vi "Log.vi"(7 "Local Variables":T2={"Core"={"Current VI"=refnum, "Close Panel on Exit?"=FALSE, "VI Name"="", "VI Path"=path ""}, "Lof File Ref"=refnum, "Log?"=FALSE, "Logging Level"=enum."Debug", "Current Case"="", "Shared Variable Address"="", "reader endpoint"="", "writer endpoint"="", "Detected Systems"=[], "Dataset"={"System Status"={"Power On Off"=FALSE, "Discharge Temp"=0.0, "Liquid Temp"=0.0, "Suction Temp"=0.0, "Ambient Temp"=0.0, "Sleep"=FALSE, "System Status"=enum."Sleep", "M1 Actuated"=FALSE, "M2 Actuated"=FALSE, "Sleep Timer"=0.0, "M1 Bin"={"Bin String"="", "Bin Color"=enum."White"}, "M2 Bin"={"Bin String"="", "Bin Color"=enum."White"}, "Discharge Pressure"=0.0, "Suction Pressure"=0.0, "Compression Ratio"=0.0, "Compressor Amps"=0.0, "Compressor Hours"=0.0, "Bypass Steps"=0, "SubCooling"=0.0, "SuperHeat"=0.0, "Serial Number"="", "EMO detected"=FALSE, "EMO Tripped"=FALSE, "Thermal cutoff"=FALSE, "Thermal cutoff 2"=FALSE, "High Pressure switch"=FALSE, "Running Time"=timestamp(0 s since 1904-01-01), "SOM Status"={"Boot Up Time"=timestamp(0 s since 1904-01-01), "Software Version"="", "CPU Usage"=0.0, "Memory Available"=0.0, "SD card free space"=0.0, "SOM Storage"=0.0}, "Cascade Extra"={"Discharge Temp High Side"=0.0, "Suction Temp High Side"=0.0, "Liquid Temp High side"=0.0, "Discharge Pressure 2"=0.0, "Suction Pressure 2"=0.0, "Low Side RPM"=0.0, "High Side RPM"=0.0}}, "M1 Status"={"Case Temp"=0.0, "Evap Temp"=0.0, "Heater %"=0.0, "EEV Steps"=0, "Set Temp"=0.0, "Feedback"=0, "Power Drive"=FALSE, "Piston Volts"=0.0, "Safe Temp"=FALSE, "Power"=FALSE, "Thermal State"=enum."Ramp Up", "Error"=FALSE, "In tollerance"=FALSE, "Head State"=enum."Disabled", "Piston Force"=0.0, "Package"="", "Dynamic SV"=0.0, "PV"=0.0, "TSD Temp"=0.0, "DC Load Watts"=0.0, "AC Load Watts"=0.0, "Intec Feedback"=0.0}, "M2 Status"={"Case Temp"=0.0, "Evap Temp"=0.0, "Heater %"=0.0, "EEV Steps"=0, "Set Temp"=0.0, "Feedback"=0, "Power Drive"=FALSE, "Piston Volts"=0.0, "Safe Temp"=FALSE, "Power"=FALSE, "Thermal State"=enum."Ramp Up", "Error"=FALSE, "In tollerance"=FALSE, "Head State"=enum."Disabled", "Piston Force"=0.0, "Package"="", "PV"=0.0, "Dynamic SV"=0.0, "TSD"=0.0, "AC Load Watts"=0.0}, "Config Data"={"Packages"={"DUT Force lbf"={" 0"=0, " 1"=0, " 2"=0, "3"=0, "4"=0, "5"=0, " 6"=0, "7"=0, "8"=0, "9"=0}, "DUT Names"={"0"="", "1"="", "2"="", "3"="", "4"="", "5"="", "6"="", "7"="", "8"="", "9"=""}}, "Heater PID"={"P"=0.0, "I"=0.0, "D"=0.0}, "Piston Settings"={"Forces Slope"=0.0, "Forces Intercept"=0.0, "Transition Force"=0.0, "Up Force"=0.0, "Diameter (mm)"=0.0, "Delay (ms)"=0.0, "Pressure Ramp Delay (ms)"=0.0}, "Safe Temps"={"Minimum"=17, "Enabled"=TRUE, "Maximum"=95}, "System Settings"={"Number of Heads"=0, "60Hz Power"=TRUE, "FTC200"=TRUE, "AutoStartup"=FALSE, "Purge"=TRUE, "Sensors"=TRUE, "HandClamp"=TRUE, "ATE"=TRUE, "Benchtop"=TRUE, "Production"=TRUE, "Refrigerant"=enum."r404a", "Handler"=TRUE, "Shuttle"=TRUE, "220V"=FALSE, "Cascade"=FALSE, "Suction Sensor"=enum."YCQB02H01", "Discharge Sensor"=enum."YCQB05H01"}, "Stepper Settings "={"Microstepping"=enum."Full", "Velocity"=8}, "Set Point Range"={"Max"=0.0, "Min"=0.0}, "Pedestal Check DeltaT"=0.0, "Ramp Delta T"=0.0, "Ramp-SS Threshold"=0.0, "SS Tolerance"=0.0, "EEV PID"={"Ramp Up Target"=0.0, "Ramp Down Target"=0.0, "Steady State Target"=0.0, "Output"={"Max"=0.0, "Min"=0.0}, "EBB and Flow Temp TH"=0.0, "Cryomode EEV Max"=0.0, "Valve minimum opening "=0.0, "Ramp Up EEV Steps"=0.0, "Ramp Down EEV Steps"=0.0, "SS EEV Steps Reset"=0.0, "EBB and Flow Tol"=0.0, "Gains"={"P"=0.0, "I"=0.0, "D"=0.0}, "Dissabled Target"=0.0, "CryoMode Gains"={"P"=0.0, "I"=0.0, "D"=0.0}, "M1 SuperHeat Setpoint"=0.0, "M2 Gains"={"P"=0.0, "I"=0.0, "D"=0.0}, "Flow Curve"=enum.""}, "Sleep Timeout"=0.0, "Bypass Values"={"Bypass Valve"=TRUE, "Flow Curve"=enum."0", "Output"={"Max"=0, "Min"=0}, "Feedback"=enum."Temperature", "Cyth Bypass"=TRUE, "PID"={"P"=0.0, "I"=0.0, "D"=0.0}, "Pressure setpoint"=0, "Cryo Temp"=0, "Superheat Setpoint"=0, "Cryo Setpoint"=0}, "Default Temp"=0.0, "InTEC"={"Enabled"=FALSE, "IP"="192.168.1.100", "Port"=5000}, "M1 TSD"={"Gain"=0.0, "Offset"=0.0, "V Offset "=0.0}, "M2 TSD"={"Gain"=0.0, "Offset"=0.0, "V Offset "=0.0}, "M1 T-Case Calibration"={"Gain"=0.0, "Offset"=0.0}, "M2 T-Case Calibration"={"Gain"=0.0, "Offset"=0.0}, "Heater PID TSD"={"P"=0.0, "I"=0.0, "D"=0.0}, "M2 Heater PID"={"P"=0.0, "I"=0.0, "D"=0.0}}}, "Network Data Down"={"M1 Commands"={"Set Temp"=20.0, "Power Drive"=FALSE, "Feedback"=1, "Package"=0, "Enable"=FALSE}, "M2 Commands"={"Set Temp"=20.0, "Power Drive"=FALSE, "Feedback"=1, "Package"=0, "Enable"=FALSE}, "System Power On Off"=FALSE, "New Data"=enum."M1 Set Point", "Stop RT"=FALSE, "Config Data"={"Packages"={"DUT Force lbf"={" 0"=0, " 1"=0, " 2"=0, "3"=0, "4"=0, "5"=0, " 6"=0, "7"=0, "8"=0, "9"=0}, "DUT Names"={"0"="", "1"="", "2"="", "3"="", "4"="", "5"="", "6"="", "7"="", "8"="", "9"=""}}, "Heater PID"={"P"=0.0, "I"=0.0, "D"=0.0}, "Piston Settings"={"Forces Slope"=0.0, "Forces Intercept"=0.0, "Transition Force"=0.0, "Up Force"=0.0, "Diameter (mm)"=0.0, "Delay (ms)"=0.0, "Pressure Ramp Delay (ms)"=0.0}, "Safe Temps"={"Minimum"=17, "Enabled"=TRUE, "Maximum"=95}, "System Settings"={"Number of Heads"=0, "60Hz Power"=TRUE, "FTC200"=TRUE, "AutoStartup"=FALSE, "Purge"=TRUE, "Sensors"=TRUE, "HandClamp"=TRUE, "ATE"=TRUE, "Benchtop"=TRUE, "Production"=TRUE, "Refrigerant"=enum."r404a", "Handler"=TRUE, "Shuttle"=TRUE, "220V"=FALSE, "Cascade"=FALSE, "Suction Sensor"=enum."YCQB02H01", "Discharge Sensor"=enum."YCQB05H01"}, "Stepper Settings "={"Microstepping"=enum."Full", "Velocity"=8}, "Set Point Range"={"Max"=0.0, "Min"=0.0}, "Pedestal Check DeltaT"=0.0, "Ramp Delta T"=0.0, "Ramp-SS Threshold"=0.0, "SS Tolerance"=0.0, "EEV PID"={"Ramp Up Target"=0.0, "Ramp Down Target"=0.0, "Steady State Target"=0.0, "Output"={"Max"=0.0, "Min"=0.0}, "EBB and Flow Temp TH"=0.0, "Cryomode EEV Max"=0.0, "Valve minimum opening "=0.0, "Ramp Up EEV Steps"=0.0, "Ramp Down EEV Steps"=0.0, "SS EEV Steps Reset"=0.0, "EBB and Flow Tol"=0.0, "Gains"={"P"=0.0, "I"=0.0, "D"=0.0}, "Dissabled Target"=0.0, "CryoMode Gains"={"P"=0.0, "I"=0.0, "D"=0.0}, "M1 SuperHeat Setpoint"=0.0, "M2 Gains"={"P"=0.0, "I"=0.0, "D"=0.0}, "Flow Curve"=enum.""}, "Sleep Timeout"=0.0, "Bypass Values"={"Bypass Valve"=TRUE, "Flow Curve"=enum."0", "Output"={"Max"=0, "Min"=0}, "Feedback"=enum."Temperature", "Cyth Bypass"=TRUE, "PID"={"P"=0.0, "I"=0.0, "D"=0.0}, "Pressure setpoint"=0, "Cryo Temp"=0, "Superheat Setpoint"=0, "Cryo Setpoint"=0}, "Default Temp"=0.0, "InTEC"={"Enabled"=FALSE, "IP"="192.168.1.100", "Port"=5000}, "M1 TSD"={"Gain"=0.0, "Offset"=0.0, "V Offset "=0.0}, "M2 TSD"={"Gain"=0.0, "Offset"=0.0, "V Offset "=0.0}, "M1 T-Case Calibration"={"Gain"=0.0, "Offset"=0.0}, "M2 T-Case Calibration"={"Gain"=0.0, "Offset"=0.0}, "Heater PID TSD"={"P"=0.0, "I"=0.0, "D"=0.0}, "M2 Heater PID"={"P"=0.0, "I"=0.0, "D"=0.0}}, "TTV Test"=FALSE, "Profile Test"=FALSE}, "IP Address"="", "Network Connection"=FALSE, "URI Directory"="", "File list in SoM"=[], "System State"=enum."Idle", "TTV Test"={"Power Seq"=[], "PS Connection"=FALSE, "OutputState"=FALSE, "Step"=0, "Current Cycle"=0}, "Profile"={"Profile Temp"=FALSE, "Profile Info"={"Start Temp"=0.0, "End Temp"=0.0, "Duration"=0.0, "dt"=0.0, "Iteration"=0}, "Current Cycle"=0}, "M1 Original Temps"=[], "M1 Mean Temps"=[], "M2 Original Temps"=[], "M2 Mean Temps"=[]} {"M2 Mean Temps" format="%#_13g"; "M2 Original Temps" format="%#_13g"; "M1 Mean Temps" format="%#_13g"; "M1 Original Temps" format="%#_13g"; "Profile"."Profile Info"."dt" format="%<%H:%M:%S>t"; "Profile"."Profile Info"."Duration" format="%<%H:%M:%S>t"; "Network Data Down"."M1 Commands"."Package" items=["CNF75XX", "CN73XX", "CN78XX", "CN88XX"]; "Network Data Down"."M1 Commands"."Feedback" items=["Evap Temp", "Case Temp"]; "Network Data Down"."M2 Commands"."Package" items=["CNF75XX", "CN73XX", "CN78XX", "CN88XX"]; "Network Data Down"."M2 Commands"."Feedback" items=["Evap Temp", "Case Temp"]; "Dataset"."System Status"."SOM Status"."Boot Up Time" format="%<%x %.3X>T"; "Dataset"."System Status"."Running Time" format="%<%x %.3X>T"; "Dataset"."M1 Status"."Feedback" items=["Evap Temp", "Case Temp", "Intec Temp", "TSD  Temp", "Autotune", "Extra"]; "Dataset"."M2 Status"."Feedback" items=["Evap Temp", "Case Temp"]}, 8 "error in (no error)":errorcluster, 11 "Log Level":T1) -> (0 "error out":errorcluster)   [LabVIEW 2019, in "GUI.lvlib"]
uses:
  GUI.lvlib
  Public Controls/GUI Variables.ctl
  Public Controls/Full Dataset.ctl
  Public Controls/Network Data Down.ctl
  Public Controls/Power Sequence.ctl
  Private Controls/Log Level.ctl
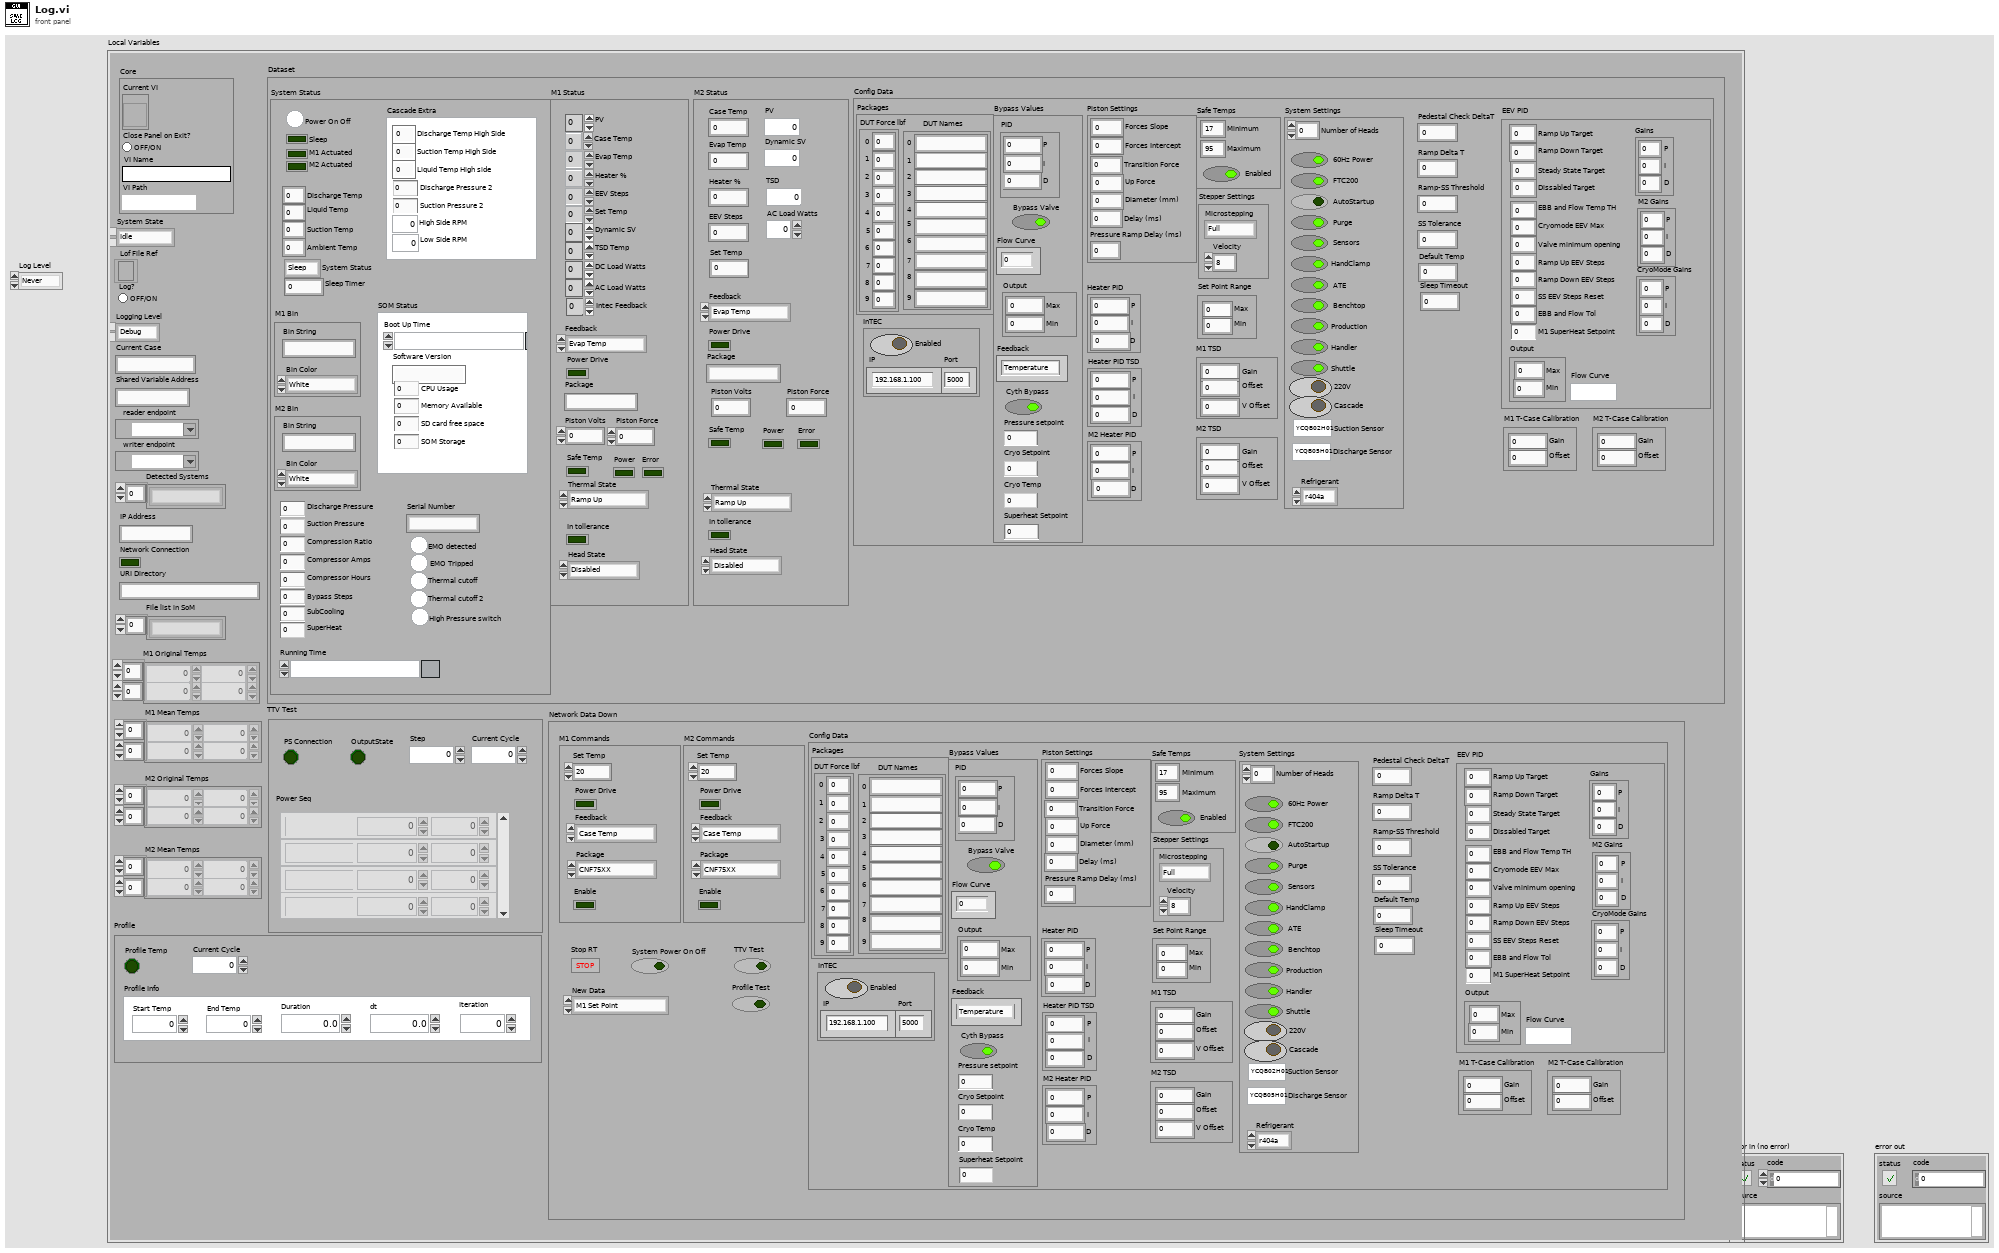
[diagram p1: front panel]
types:
  T1 = typedef "GUI.lvlib/Log Level.ctl" = enum16{"Never", "Debug", "Info", "Critical"}
  T2 = typedef "GUI.lvlib/GUI Variables.ctl" = cluster{"Core":cluster{"Current VI":refnum<vi>, "Close Panel on Exit?":bool, "VI Name":string, "VI Path":path}, "Lof File Ref":refnum<file>, "Log?":bool, "Logging Level":enum16{"Never", "Debug", "Info", "Critical"}, "Current Case":string, "Shared Variable Address":string, "reader endpoint":refnum<k21>, "writer endpoint":refnum<k21>, "Detected Systems":string[], "Dataset":T3, "Network Data Down":T4, "IP Address":string, "Network Connection":bool, "URI Directory":string, "File list in SoM":string[], "System State":enum16{"Idle", "Running"}, "TTV Test":cluster{"Power Seq":T5, "PS Connection":bool, "OutputState":bool, "Step":i32, "Current Cycle":i32}, "Profile":cluster{"Profile Temp":bool, "Profile Info":cluster{"Start Temp":dbl, "End Temp":dbl, "Duration":dbl, "dt":dbl, "Iteration":i32}, "Current Cycle":i32}, "M1 Original Temps":dbl[][], "M1 Mean Temps":dbl[][], "M2 Original Temps":dbl[][], "M2 Mean Temps":dbl[][]}
  T3 = typedef "GUI.lvlib/Full Dataset.ctl" = cluster{"System Status":cluster{"Power On Off":bool, "Discharge Temp":dbl, "Liquid Temp":dbl, "Suction Temp":dbl, "Ambient Temp":dbl, "Sleep":bool, "System Status":enum16{"Sleep", "Run"}, "M1 Actuated":bool, "M2 Actuated":bool, "Sleep Timer":dbl, "M1 Bin":cluster{"Bin String":string, "Bin Color":enum16{"Black", "White", "Red", "Green", "Blue", "Cyan", "Amber"}}, "M2 Bin":cluster{"Bin String":string, "Bin Color":enum16{"Black", "White", "Red", "Green", "Blue", "Cyan", "Amber"}}, "Discharge Pressure":dbl, "Suction Pressure":dbl, "Compression Ratio":dbl, "Compressor Amps":dbl, "Compressor Hours":dbl, "Bypass Steps":u16, "SubCooling":dbl, "SuperHeat":dbl, "Serial Number":string, "EMO detected":bool, "EMO Tripped":bool, "Thermal cutoff":bool, "Thermal cutoff 2":bool, "High Pressure switch":bool, "Running Time":timestamp, "SOM Status":cluster{"Boot Up Time":timestamp, "Software Version":string, "CPU Usage":dbl, "Memory Available":dbl, "SD card free space":dbl, "SOM Storage":dbl}, "Cascade Extra":cluster{"Discharge Temp High Side":dbl, "Suction Temp High Side":dbl, "Liquid Temp High side":dbl, "Discharge Pressure 2":dbl, "Suction Pressure 2":dbl, "Low Side RPM":dbl, "High Side RPM":dbl}}, "M1 Status":cluster{"Case Temp":dbl, "Evap Temp":dbl, "Heater %":dbl, "EEV Steps":u32, "Set Temp":dbl, "Feedback":u8, "Power Drive":bool, "Piston Volts":dbl, "Safe Temp":bool, "Power":bool, "Thermal State":enum16{"Ramp Up", "Ramp Down", "Steady State", "Ebb and Flow", "Up", "Under Load", "Cryo Mode"}, "Error":bool, "In tollerance":bool, "Head State":enum16{"Disabled", "Run", "Error"}, "Piston Force":dbl, "Package":string, "Dynamic SV":dbl, "PV":dbl, "TSD Temp":dbl, "DC Load Watts":dbl, "AC Load Watts":dbl, "Intec Feedback":dbl}, "M2 Status":cluster{"Case Temp":dbl, "Evap Temp":dbl, "Heater %":dbl, "EEV Steps":u32, "Set Temp":dbl, "Feedback":u8, "Power Drive":bool, "Piston Volts":dbl, "Safe Temp":bool, "Power":bool, "Thermal State":enum16{"Ramp Up", "Ramp Down", "Steady State", "Ebb and Flow", "Up"}, "Error":bool, "In tollerance":bool, "Head State":enum16{"Disabled", "Run", "Error"}, "Piston Force":dbl, "Package":string, "PV":dbl, "Dynamic SV":dbl, "TSD":dbl, "AC Load Watts":dbl}, "Config Data":cluster{"Packages":cluster{"DUT Force lbf":cluster{" 0":u32, " 1":u32, " 2":u32, "3":u32, "4":u32, "5":u32, " 6":u32, "7":u32, "8":u32, "9":u32}, "DUT Names":cluster{"0":string, "1":string, "2":string, "3":string, "4":string, "5":string, "6":string, "7":string, "8":string, "9":string}}, "Heater PID":cluster{"P":dbl, "I":dbl, "D":dbl}, "Piston Settings":cluster{"Forces Slope":dbl, "Forces Intercept":dbl, "Transition Force":dbl, "Up Force":dbl, "Diameter (mm)":dbl, "Delay (ms)":dbl, "Pressure Ramp Delay (ms)":dbl}, "Safe Temps":cluster{"Minimum":i32, "Enabled":bool, "Maximum":i32}, "System Settings":cluster{"Number of Heads":i32, "60Hz Power":bool, "FTC200":bool, "AutoStartup":bool, "Purge":bool, "Sensors":bool, "HandClamp":bool, "ATE":bool, "Benchtop":bool, "Production":bool, "Refrigerant":enum16{"r404a", "r507", "r508", "r410a", "r134a"}, "Handler":bool, "Shuttle":bool, "220V":bool, "Cascade":bool, "Suction Sensor":enum16{"YCQB02H01", "YCQB02L01", "Carel"}, "Discharge Sensor":enum16{"YCQB05H01", "YCQB05L01", "Carel"}}, "Stepper Settings ":cluster{"Microstepping":enum16{"Full", "Half", "Quarter", "1/16th"}, "Velocity":u8}, "Set Point Range":cluster{"Max":dbl, "Min":dbl}, "Pedestal Check DeltaT":dbl, "Ramp Delta T":dbl, "Ramp-SS Threshold":dbl, "SS Tolerance":dbl, "EEV PID":cluster{"Ramp Up Target":dbl, "Ramp Down Target":dbl, "Steady State Target":dbl, "Output":cluster{"Max":dbl, "Min":dbl}, "EBB and Flow Temp TH":dbl, "Cryomode EEV Max":dbl, "Valve minimum opening ":dbl, "Ramp Up EEV Steps":dbl, "Ramp Down EEV Steps":dbl, "SS EEV Steps Reset":dbl, "EBB and Flow Tol":dbl, "Gains":cluster{"P":dbl, "I":dbl, "D":dbl}, "Dissabled Target":dbl, "CryoMode Gains":cluster{"P":dbl, "I":dbl, "D":dbl}, "M1 SuperHeat Setpoint":dbl, "M2 Gains":cluster{"P":dbl, "I":dbl, "D":dbl}, "Flow Curve":enum16{""}}, "Sleep Timeout":dbl, "Bypass Values":cluster{"Bypass Valve":bool, "Flow Curve":enum16{"0", "1"}, "Output":cluster{"Max":u32, "Min":u32}, "Feedback":enum16{"Temperature", "Pressure", "Superheat", "Pressure 2.0"}, "Cyth Bypass":bool, "PID":cluster{"P":dbl, "I":dbl, "D":dbl}, "Pressure setpoint":i16, "Cryo Temp":i16, "Superheat Setpoint":i16, "Cryo Setpoint":i16}, "Default Temp":dbl, "InTEC":cluster{"Enabled":bool, "IP":string, "Port":u16}, "M1 TSD":cluster{"Gain":dbl, "Offset":dbl, "V Offset ":dbl}, "M2 TSD":cluster{"Gain":dbl, "Offset":dbl, "V Offset ":dbl}, "M1 T-Case Calibration":cluster{"Gain":dbl, "Offset":dbl}, "M2 T-Case Calibration":cluster{"Gain":dbl, "Offset":dbl}, "Heater PID TSD":cluster{"P":dbl, "I":dbl, "D":dbl}, "M2 Heater PID":cluster{"P":dbl, "I":dbl, "D":dbl}}}
  T4 = typedef "GUI.lvlib/Network Data Down.ctl" = cluster{"M1 Commands":cluster{"Set Temp":dbl, "Power Drive":bool, "Feedback":u8, "Package":u16, "Enable":bool}, "M2 Commands":cluster{"Set Temp":dbl, "Power Drive":bool, "Feedback":u8, "Package":u16, "Enable":bool}, "System Power On Off":bool, "New Data":enum16{"M1 Set Point", "M1 Power Drive", "M1 Feedback", "M1 Package", "M1 Enable", "M2 Set Point", "M2 Power Drive", "M2 Feedback", "M2 Package", "M2 Enable", "System Power", "Config Data", "TTV Test", "Profile Test", "Stop RT"}, "Stop RT":bool, "Config Data":cluster{"Packages":cluster{"DUT Force lbf":cluster{" 0":u32, " 1":u32, " 2":u32, "3":u32, "4":u32, "5":u32, " 6":u32, "7":u32, "8":u32, "9":u32}, "DUT Names":cluster{"0":string, "1":string, "2":string, "3":string, "4":string, "5":string, "6":string, "7":string, "8":string, "9":string}}, "Heater PID":cluster{"P":dbl, "I":dbl, "D":dbl}, "Piston Settings":cluster{"Forces Slope":dbl, "Forces Intercept":dbl, "Transition Force":dbl, "Up Force":dbl, "Diameter (mm)":dbl, "Delay (ms)":dbl, "Pressure Ramp Delay (ms)":dbl}, "Safe Temps":cluster{"Minimum":i32, "Enabled":bool, "Maximum":i32}, "System Settings":cluster{"Number of Heads":i32, "60Hz Power":bool, "FTC200":bool, "AutoStartup":bool, "Purge":bool, "Sensors":bool, "HandClamp":bool, "ATE":bool, "Benchtop":bool, "Production":bool, "Refrigerant":enum16{"r404a", "r507", "r508", "r410a", "r134a"}, "Handler":bool, "Shuttle":bool, "220V":bool, "Cascade":bool, "Suction Sensor":enum16{"YCQB02H01", "YCQB02L01", "Carel"}, "Discharge Sensor":enum16{"YCQB05H01", "YCQB05L01", "Carel"}}, "Stepper Settings ":cluster{"Microstepping":enum16{"Full", "Half", "Quarter", "1/16th"}, "Velocity":u8}, "Set Point Range":cluster{"Max":dbl, "Min":dbl}, "Pedestal Check DeltaT":dbl, "Ramp Delta T":dbl, "Ramp-SS Threshold":dbl, "SS Tolerance":dbl, "EEV PID":cluster{"Ramp Up Target":dbl, "Ramp Down Target":dbl, "Steady State Target":dbl, "Output":cluster{"Max":dbl, "Min":dbl}, "EBB and Flow Temp TH":dbl, "Cryomode EEV Max":dbl, "Valve minimum opening ":dbl, "Ramp Up EEV Steps":dbl, "Ramp Down EEV Steps":dbl, "SS EEV Steps Reset":dbl, "EBB and Flow Tol":dbl, "Gains":cluster{"P":dbl, "I":dbl, "D":dbl}, "Dissabled Target":dbl, "CryoMode Gains":cluster{"P":dbl, "I":dbl, "D":dbl}, "M1 SuperHeat Setpoint":dbl, "M2 Gains":cluster{"P":dbl, "I":dbl, "D":dbl}, "Flow Curve":enum16{""}}, "Sleep Timeout":dbl, "Bypass Values":cluster{"Bypass Valve":bool, "Flow Curve":enum16{"0", "1"}, "Output":cluster{"Max":u32, "Min":u32}, "Feedback":enum16{"Temperature", "Pressure", "Superheat", "Pressure 2.0"}, "Cyth Bypass":bool, "PID":cluster{"P":dbl, "I":dbl, "D":dbl}, "Pressure setpoint":i16, "Cryo Temp":i16, "Superheat Setpoint":i16, "Cryo Setpoint":i16}, "Default Temp":dbl, "InTEC":cluster{"Enabled":bool, "IP":string, "Port":u16}, "M1 TSD":cluster{"Gain":dbl, "Offset":dbl, "V Offset ":dbl}, "M2 TSD":cluster{"Gain":dbl, "Offset":dbl, "V Offset ":dbl}, "M1 T-Case Calibration":cluster{"Gain":dbl, "Offset":dbl}, "M2 T-Case Calibration":cluster{"Gain":dbl, "Offset":dbl}, "Heater PID TSD":cluster{"P":dbl, "I":dbl, "D":dbl}, "M2 Heater PID":cluster{"P":dbl, "I":dbl, "D":dbl}}, "TTV Test":bool, "Profile Test":bool}
  T5 = typedef "GUI.lvlib/Power Sequence.ctl" = cluster{"Duration":i32, "Head Load(W)":u32, "Name":string}[]
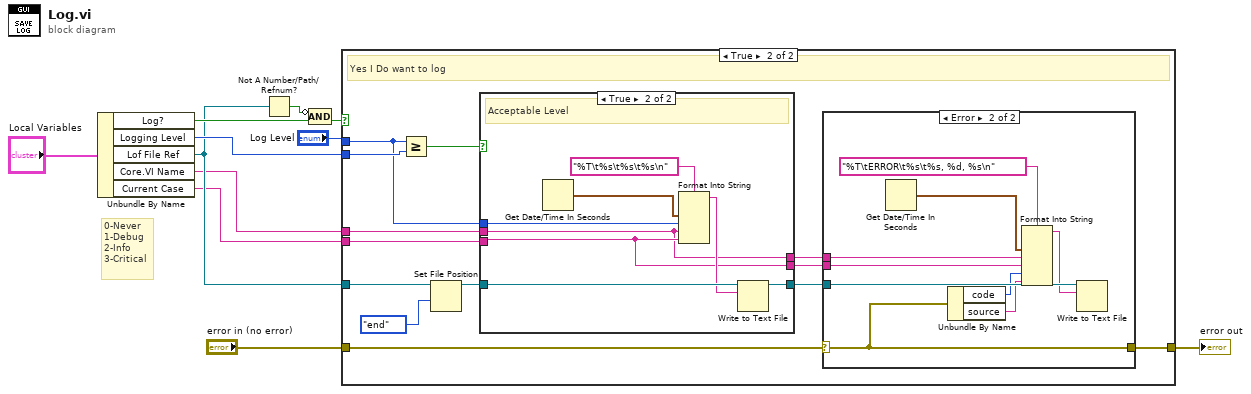
[diagram p0: block diagram]
diagram:
  # "0-Never\n1-Debug\n2-Info\n3-Critical"
  n1 = Unbundle By Name("Local Variables") -> ("Log?"=w9:bool, "Logging Level"=w8:enum16{"Never", "Debug", "Info", "Critical"}, "Lof File Ref"=w5:refnum<file>, "Core.VI Name"=w4:string, "Current Case"=w3:string)
  n2 = Not A Number/Path/Refnum?(number/path/refnum=w5) -> (NaN/Path/Refnum?=w6:bool)
  n3 = Compound Arithmetic op=AND(invert w6, w9) -> (w7:bool)
  n4 = case shown="True" w7 {
    tunnel: [w12 w23] -> w11
    tunnel: "error in (no error)" -> [w12 w16]
    tunnel: w5 -> [_ w19]
    tunnel: w8 -> [_ w25]
    tunnel: "Log Level" -> [_ w21]
    tunnel: w4 -> [_ w15]
    tunnel: w3 -> [_ w14]
    frame False {
      # "No I do not want to log"
    }
    frame True {
      # "Yes I Do want to log"
      n5 = Greater Or Equal?(x=w21, y=w25) -> (x >= y?=w24:bool)
      n6 = Set File Position(refnum=w19, from (0:start)=enum16{"start", "end", "current"}."end") -> (refnum out=w18:refnum<file>)  [unwired: 2 in, 1 out]
      n7 = case shown="True" w24 {
        tunnel: w18 -> [w38 w46]
        tunnel: [w38 w45] -> w22
        tunnel: w21 -> [_ w43]
        tunnel: [w37 w40] -> w20
        tunnel: w15 -> [w36 w39]
        tunnel: w14 -> [w37 w40]
        tunnel: [w36 w39] -> w13
        frame False {
          # "Wrong level"
        }
        frame True {
          # "Acceptable Level"
          n8 = Get Date/Time In Seconds() -> (seconds since 1Jan1904=w42:timestamp)
          n9 = Format Into String(format string="%T\t%s\t%s\t%s\n", w42, w43, w39, w40) -> (resulting string=w41:string)  [unwired: 2 in, 1 out]
          n10 = Write to Text File(file (use dialog)=w46, text=w41) -> (refnum out=w45:refnum<file>)  [unwired: 2 in, 2 out]
        }
      }
      n11 = case shown="Error" w16 {
        selector: w16 -> [w26 w31]
        tunnel: [w26 w31] -> w23
        tunnel: w22 -> [_ w35]
        tunnel: w20 -> [_ w28]
        tunnel: w13 -> [_ w27]
        frame No Error {
        }
        frame Error {
          n12 = Get Date/Time In Seconds() -> (seconds since 1Jan1904=w34:timestamp)
          n13 = Unbundle By Name(w31) -> ("code"=w30:i32, "source"=w29:string)
          n14 = Format Into String(format string="%T\tERROR\t%s\t%s, %d, %s\n", w34, w27, w28, w30, w29) -> (resulting string=w32:string)  [unwired: 2 in, 1 out]
          n15 = Write to Text File(file (use dialog)=w35, text=w32) -> ()  [unwired: 2 in, 3 out]
        }
      }
    }
  }
  "error out" <- w11
